vi "Init Module.vi"(8 "error in (no error)":errorcluster, 11 "Singleton Module Admin in":refnum<class "Delacor_lib_QMH_Module Admin.lvclass">) -> (0 "error out":errorcluster, 2 "Power Supply Request Events":T1, 3 "Singleton Module Admin out":refnum<class "Delacor_lib_QMH_Module Admin.lvclass">)   [LabVIEW 2025, in "Power Supply.lvlib"]
doc: "Initialize the module by creating Broadcast Events, Request Events, and synchronization rendezvous.\n_____\nBased on Delacor QMH Project Template 3.1.0.34.\n\n<b>Note:</b> This VI was modified by the <b>Validate DQMH Module</b> tool to add the 'Show Main VI Diagram on Init' functionality included in DQMH 6.1."
uses:
  Power Supply.lvlib
  <vilib>/Delacor/Delacor QMH/Libraries/Module Admin_class/Delacor_lib_QMH_Module Admin.lvclass
  Stop Argument--cluster.ctl
  Request Events--cluster.ctl
  Get Module Execution Status Argument--cluster.ctl
  Show Diagram Argument--cluster.ctl
  Show Panel Argument--cluster.ctl
  Hide Panel Argument--cluster.ctl
  <vilib>/MGI/Panel Manager/Panel/Panel/Panel.lvclass
  Change Panel Argument--cluster.ctl
  Set Current SP Argument--cluster.ctl
  Set Voltage SP Argument--cluster.ctl
  Set Power SP Argument--cluster.ctl
  Set Power Supply Plugin Argument--cluster.ctl
  DC Output--enum.ctl
  Set DC Output Argument--cluster.ctl
  Sleep Connection Helper Loop Argument--cluster.ctl
  Connect Argument--cluster.ctl
  Disconnect Argument--cluster.ctl
  Function Generator State--cluster.ctl
  Set Function Generator State Argument--cluster.ctl
  Wake Connection Helper Loop Argument--cluster.ctl
  Set DC Current SP Argument--cluster.ctl
  Set DC Voltage SP Argument--cluster.ctl
  Set DC Power SP Argument--cluster.ctl
  Set DC Output SP Argument--cluster.ctl
  Function Generator Parameters--cluster.ctl
  Set Function Generator Parameters Argument--cluster.ctl
  Set Function Generator Parameters SP Argument--cluster.ctl
  Set Function Generator State SP Argument--cluster.ctl
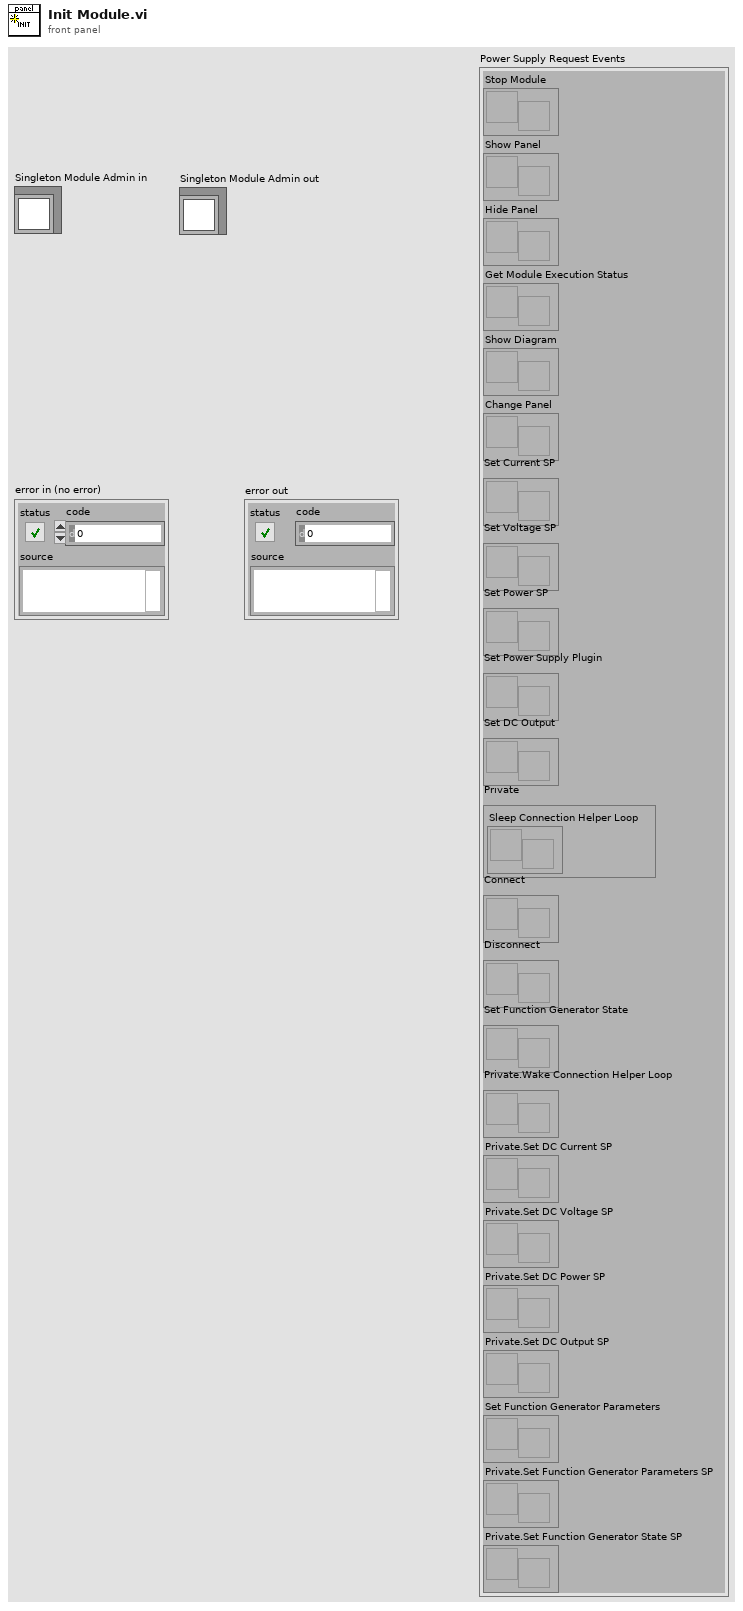
[diagram p1: front panel]
types:
  T1 = typedef "Power Supply.lvlib/Request Events--cluster.ctl" = cluster{"Stop Module":refnum<user-event>, "Show Panel":refnum<user-event>, "Hide Panel":refnum<user-event>, "Get Module Execution Status":refnum<user-event>, "Show Diagram":refnum<user-event>, "Change Panel":refnum<user-event>, "Set Current SP":refnum<user-event>, "Set Voltage SP":refnum<user-event>, "Set Power SP":refnum<user-event>, "Set Power Supply Plugin":refnum<user-event>, "Set DC Output":refnum<user-event>, "Private":cluster{"Sleep Connection Helper Loop":refnum<user-event>}, "Connect":refnum<user-event>, "Disconnect":refnum<user-event>, "Set Function Generator State":refnum<user-event>, "Private.Wake Connection Helper Loop":refnum<user-event>, "Private.Set DC Current SP":refnum<user-event>, "Private.Set DC Voltage SP":refnum<user-event>, "Private.Set DC Power SP":refnum<user-event>, "Private.Set DC Output SP":refnum<user-event>, "Set Function Generator Parameters":refnum<user-event>, "Private.Set Function Generator Parameters SP":refnum<user-event>, "Private.Set Function Generator State SP":refnum<user-event>}
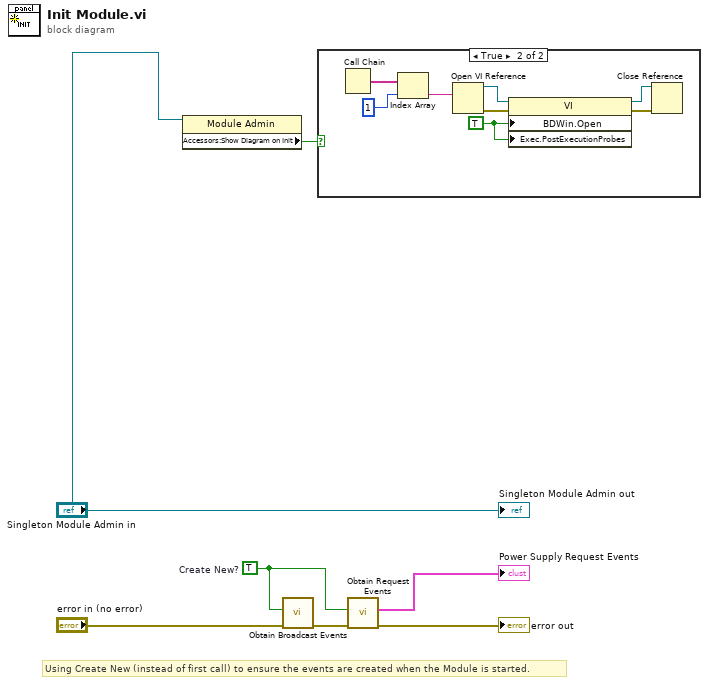
[diagram p0: block diagram]
diagram:
  w4 = TRUE  # Create New?
  # "Using Create New (instead of first call) to ensure the events are created when the Module is started."
  n1 = property class="Module Admin"(reference="Singleton Module Admin in") -> ("Accessors:Show Diagram on Init"=w1:bool)  [unwired: 1 in, 2 out]
  n2 = call "Obtain Broadcast Events.vi"("error in (no error)"="error in (no error)", "Create New?"=w4) -> ("error out"=w7:errorcluster)  [unwired: 8 in, 1 out]
  n3 = case shown="True" w1 {
    frame False {
    }
    frame True {
      w11 = TRUE ("Block Diagram Window:Open")
      n4 = Call Chain() -> (call chain=w15:string[])
      n5 = Index Array(array=w15, index=1) -> (element=w8:string)
      n6 = Open VI Reference(vi path=w8) -> (vi reference=w12:refnum<vi>, error out=w13:errorcluster)  [unwired: 5 in]
      n7 = property class="VI"(reference=w12, error in=w13, "BDWin.Open"=w11, "Exec.PostExecutionProbes"=w11) -> (reference out=w9:refnum<vi>, error out=w10:errorcluster)
      n8 = Close Reference(reference=w9, error in (no error)=w10) -> ()  [unwired: 1 out]
    }
  }
  n9 = call "Obtain Request Events.vi"("error in (no error)"=w7, "Create New?"=w4) -> ("error out"=→"error out":errorcluster, "Power Supply Request Events"=→"Power Supply Request Events":T1)  [unwired: 8 in]
  "Singleton Module Admin out" <- "Singleton Module Admin in"
